vi "Set Acq Status Event.vi"(8 "error in (no error)":errorcluster, 11 "statusEvent":u32) -> (0 "error out":errorcluster, 2 "function return":u32, 3 "statusEvent out":u32)   [LabVIEW 2014, in "atmcd32d.lvlib"]
doc: "unsigned int WINAPI SetAcqStatusEvent(HANDLE statusEvent);"
uses:
  atmcd32d.lvlib
  atmcd32d.dll
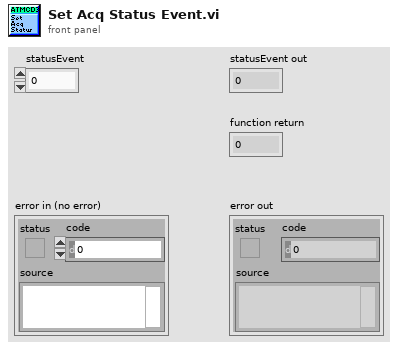
[diagram p1: front panel]
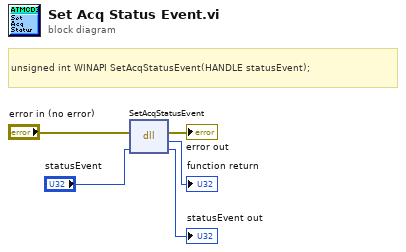
[diagram p0: block diagram]
diagram:
  # "unsigned int WINAPI SetAcqStatusEvent(HANDLE statusEvent);"
  n1 = dll-call lib="C:/Users/Bakir/Documents/Lambda2-Testing/lib/Andorlib/atmcd32d.*" fn="SetAcqStatusEvent"(error in="error in (no error)", "statusEvent"="statusEvent") -> (error out=→"error out":errorcluster, →"function return":u32, "statusEvent"=→"statusEvent out":u32)  [unwired: 2 in, 1 out]
